vi "moveXYToInitialPos.vi"(8 "error in":errorcluster) -> (0 "error out":errorcluster)   [LabVIEW 2014]
doc: "André Romero - 2023\nandretec@ifsc.usp.br\nIFSC - USP"
uses:
  Global Motors.vi
panel:
  out "pfAccn":sgl
  out "pfMaxVel":sgl
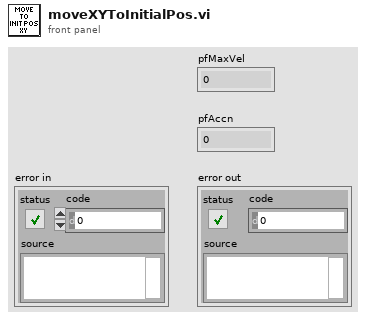
[diagram p1: front panel]
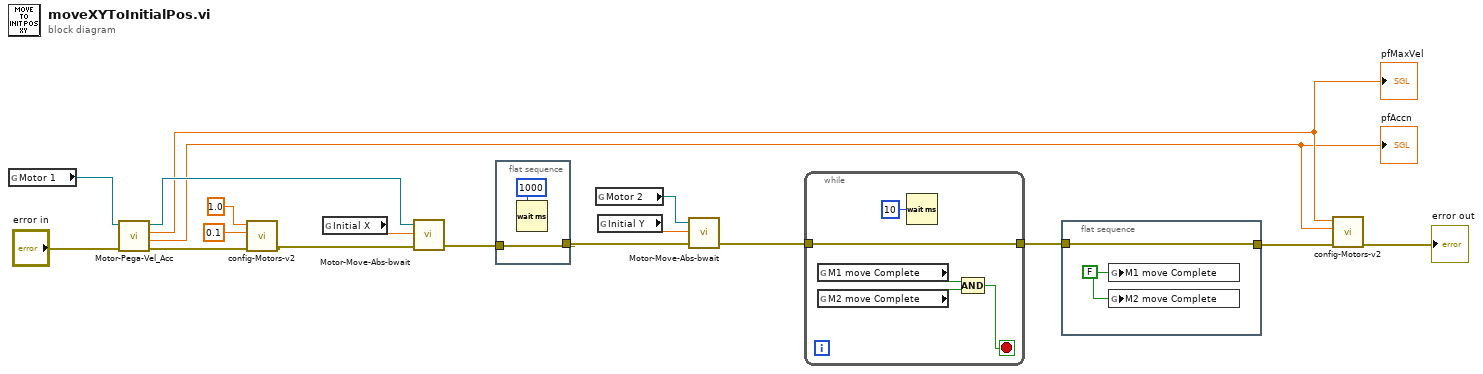
[diagram p0: block diagram]
diagram:
  n1 = global read "Global Motors.vi" "Motor 1"() -> (w8:refnum<k7>)
  n2 = call "Motor-Pega-Vel_Acc.vi"("error out"="error in", "MG17Motor in"=w8) -> ("error out 2"=w5:errorcluster, "pfAccn"=w1:sgl, "pfMaxVel"=w2:sgl, "MG17Motor out"=w7:refnum<k7>)  [unwired: 2 in]
  "pfMaxVel" <- w2
  "pfAccn" <- w1
  n3 = call "config-Motors-v2.vi"("error in"=w5, "Acc"=0.1, "Velocity"=sgl 1.0) -> ("error out"=w11:errorcluster)  [unwired: 8 in]
  n4 = global read "Global Motors.vi" "Initial X"() -> (w12:dbl)
  n5 = call "Motor-Move-Abs-bwait.vi"("error"=w11, "Posição"=w12, "MG17Motor A"=w7) -> ("error out"=w17:errorcluster)  [unwired: 1 in, 1 out]
  n6 = flat-sequence {
    tunnel: w17 -> [w20]
    tunnel: [w20] -> w18
    frame #0 {
      n7 = Wait (ms)(milliseconds to wait=u32 1000) -> ()  [unwired: 1 out]
    }
  }
  n8 = global read "Global Motors.vi" "Motor 2"() -> (w13:refnum<k7>)
  n9 = global read "Global Motors.vi" "Initial Y"() -> (w14:dbl)
  n10 = call "Motor-Move-Abs-bwait.vi"("error"=w18, "Posição"=w14, "MG17Motor A"=w13) -> ("error out"=w15:errorcluster)  [unwired: 1 in, 1 out]
  n11 = while {
    tunnel: w15 -> [w25]
    tunnel: [w25] -> w16
    stop <- w22 stop-if-true
    n12 = global read "Global Motors.vi" "M1 move Complete"() -> (w24:bool)
    n13 = global read "Global Motors.vi" "M2 move Complete"() -> (w23:bool)
    n14 = Wait (ms)(milliseconds to wait=u32 10) -> ()  [unwired: 1 out]
    n15 = Compound Arithmetic op=AND(w24, w23) -> (w22:bool)
  }
  n16 = flat-sequence {
    tunnel: w16 -> [w26]
    tunnel: [w26] -> w4
    frame #0 {
      w27 = FALSE ("M1 move Complete")
      n17 = global write "Global Motors.vi" "M1 move Complete"(w27) -> ()
      n18 = global write "Global Motors.vi" "M2 move Complete"(w27) -> ()
    }
  }
  n19 = call "config-Motors-v2.vi"("error in"=w4, "Acc"=w1, "Velocity"=w2) -> ("error out"=→"error out":errorcluster)  [unwired: 8 in]
